vi "wait_for_pattern.vi"(0 "serial in":refnum<visa-resource-name>, 1 "error in (no error)":errorcluster) -> (3 "pattern string":string, 4 "pattern detected":bool, 5 "serial out":refnum<visa-resource-name>, 6 "error out":errorcluster)   [LabVIEW 2016]
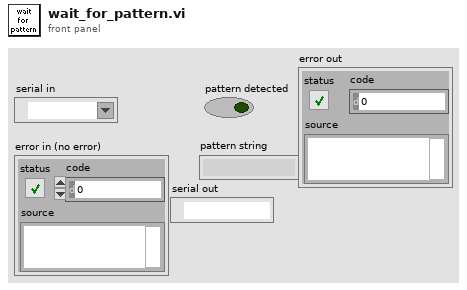
[diagram p1: front panel]
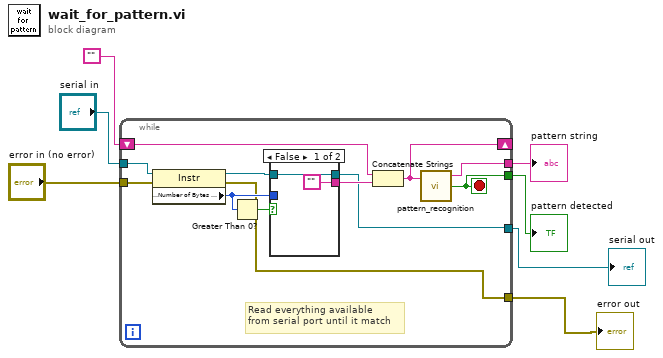
[diagram p0: block diagram]
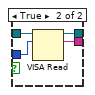
[diagram p2: hidden frame]
diagram:
  n1 = while {
    tunnel: "serial in" -> [w16]
    shift-right: [w13] -> _
    shift-left: "" -> [w15]
    tunnel: [w12] -> w5
    tunnel: [w11] -> w6
    tunnel: "error in (no error)" -> [w10]
    tunnel: [w9] -> w2
    tunnel: [w8] -> w1
    stop <- w12 stop-if-true
    # "Read everything available\nfrom serial port until it match"
    n2 = property class="Instr"(reference=w16, error in=w10) -> (reference out=w19:refnum<visa-resource-name>, error out=w8:errorcluster, "Serial Settings:Number of Bytes at Serial Port"=w17:u32)
    n3 = Greater Than 0?(x=w17) -> (x > 0?=w18:bool)
    n4 = case shown="False" w18 {
      tunnel: w19 -> [w20 w25]
      tunnel: ["" w24] -> w14
      tunnel: w17 -> [_ w23]
      tunnel: [w20 w22] -> w9
      frame False {
      }
      frame True {
        n5 = VISA Read(VISA resource name=w25, byte count=w23) -> (VISA resource name out=w22:refnum<visa-resource-name>, read buffer=w24:string)  [unwired: 1 in, 2 out]
      }
    }
    n6 = Concatenate Strings(w15, w14) -> (w13:string)
    n7 = call "pattern_recognition.vi"("read buffer in"=w13) -> ("read buffer out"=w11:string, "Boolean"=w12:bool)  [unwired: 2 in]
  }
  "pattern string" <- w6
  "pattern detected" <- w5
  "serial out" <- w2
  "error out" <- w1
